vi "Dependencies Array To ListBox.vi"(11 "All Dependencies Properties":T1[](array[typedef])) -> (3 "Array":string[][](array[string]))   [LabVIEW 2019, in "Dependencies.lvclass"]
uses:
  Dependencies.lvclass
  XML Controls/Dependencies Properties.ctl
  XML Controls/Path Cluster.ctl
  XML Controls/Supported Targets.ctl
  Configuration Tool.lvlib
  VeriStand Custom Device XML Parser.lvlib
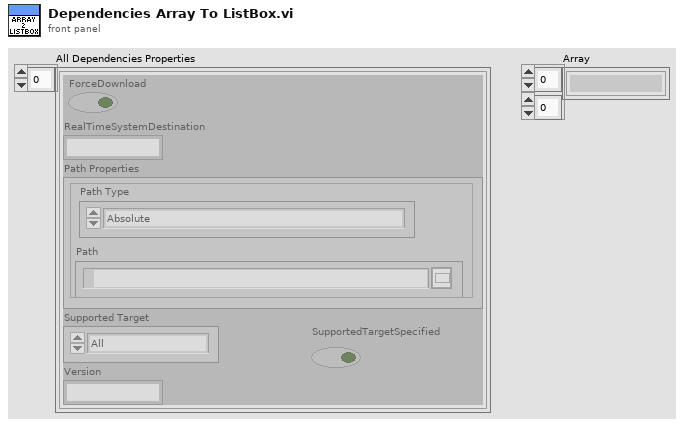
[diagram p1: front panel]
types:
  T1 = typedef "VeriStand Custom Device XML Parser.lvlib/Dependencies Properties.ctl" = cluster{"ForceDownload":bool, "RealTimeSystemDestination":string, "Path Properties":T2, "Supported Target":T3, "Version":string, "SupportedTargetSpecified":bool}
  T2 = typedef "VeriStand Custom Device XML Parser.lvlib/Path Cluster.ctl" = cluster{"Path":path, "Path Type":enum16{"Absolute", "To Base", "To Common Doc Dir", "To Application Data Dir"}}
  T3 = typedef "VeriStand Custom Device XML Parser.lvlib/Supported Targets.ctl" = enum16{"All", "Pharlap", "VxWorks", "Windows", "Linux_32_ARM", "Linux_x64", "PharlapWindows", "PharlapVxWorks", "VxWorksWindows"}
  T4 = enum16{"Absolute", "To Base", "To Common Doc Dir", "To Application Data Dir"}
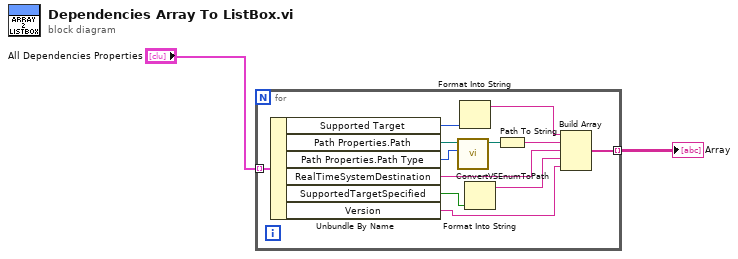
[diagram p0: block diagram]
diagram:
  n1 = for {
    tunnel: "All Dependencies Properties" -> [w14] mode=indexing
    tunnel: [w6] -> w2 mode=indexing
    n2 = Unbundle By Name(w14) -> ("Supported Target"=w13:T3, "Path Properties.Path"=w12:path, "Path Properties.Path Type"=w11:T4, "RealTimeSystemDestination"=w7:string, "SupportedTargetSpecified"=w5:bool, "Version"=w3:string)
    n3 = call "ConvertVSEnumToPath.vi"("Source.Path Type"=w11, "Path In"=w12) -> ("appended path"=w10:path)  [unwired: 9 in]
    n4 = Format Into String(w13) -> (resulting string=w9:string)  [unwired: 3 in, 1 out]
    n5 = Format Into String(w5) -> (resulting string=w4:string)  [unwired: 3 in, 1 out]
    n6 = Path To String(path=w10) -> (string=w8:string)
    n7 = Build Array(w9, w8, w7, w4, w3) -> (w6:string[])
  }
  "Array" <- w2
